vi "Mass Compile LabVIEW Tool__jki_lib_application_control -- VI Tester.vi"(8 "error in (no error)":errorcluster, 10 "Product Folders":path[](array[path]), 11 "Product Name":string) -> (0 "error out":errorcluster)   [LabVIEW 2011]
doc: "This VI self-mass compiles an installed LabVIEW Tool. It should be run by a tool, during its start-up process."
panel:
  # "Copyright © 2006-2009 James Kring, Inc. All rights reserved.\n\nAuthor: Jim Kring <jim.kring@jameskring.comm>\n\nThis library is provided \"AS IS\" , WITHOUT WARRANTIES OR \nCONDITIONS OF ANY KIND, either express or implied.\n\nJames Kring, Inc. -- http://www.jameskring.com"
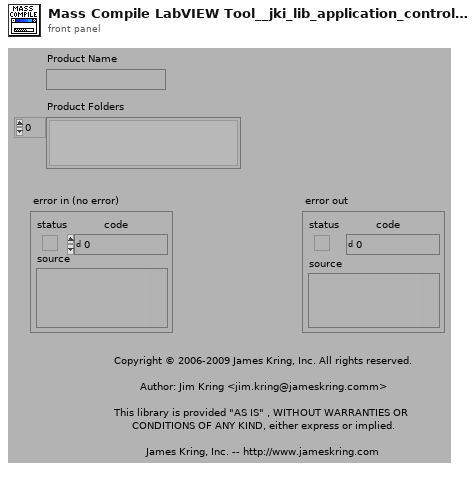
[diagram p1: front panel]
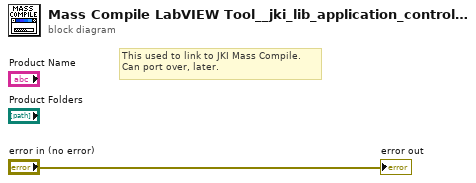
[diagram p0: block diagram]
diagram:
  # "This used to link to JKI Mass Compile.\nCan port over, later."
  "error out" <- "error in (no error)"
